vi "Get Number of Channels.vi"(8 "error in (no error)":errorcluster, 11 "Refnum in":refnum<k21>) -> (0 "error out":errorcluster, 3 "Number of Channels":i32)   [LabVIEW 2026, in "Acquisition.lvlib"]
uses:
  Acquisition.lvlib
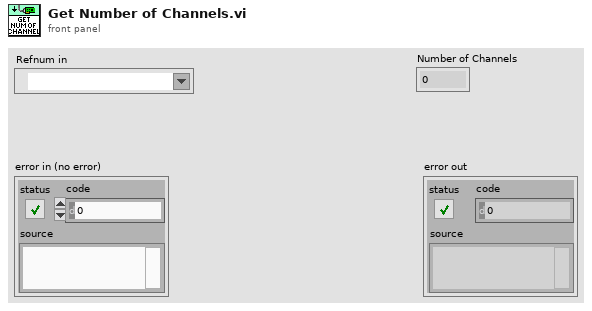
[diagram p1: front panel]
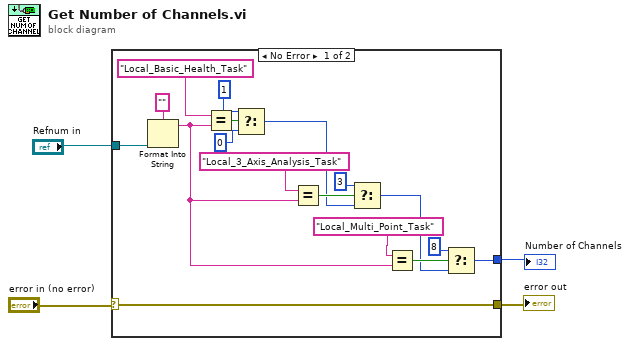
[diagram p0: block diagram]
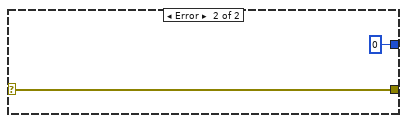
[diagram p2: hidden frame]
diagram:
  n1 = case shown="No Error" "error in (no error)" {
    selector: "error in (no error)" -> [w6 w23]
    tunnel: "Refnum in" -> [w17 _]
    tunnel: [w7 0] -> w3
    tunnel: [w6 w23] -> w1
    frame No Error {
      n2 = Format Into String(format string="", w17) -> (resulting string=w9:string)  [unwired: 2 in, 1 out]
      n3 = Equal?(x="Local_Basic_Health_Task" ("format string"), y=w9) -> (x = y?=w18:bool)
      n4 = Select(t=1, s=w18, f=0) -> (s? t:f=w13:i32)
      n5 = Equal?(x="Local_3_Axis_Analysis_Task" ("format string"), y=w9) -> (x = y?=w14:bool)
      n6 = Select(t=3, s=w14, f=w13) -> (s? t:f=w8:i32)
      n7 = Equal?(x="Local_Multi_Point_Task" ("format string"), y=w9) -> (x = y?=w11:bool)
      n8 = Select(t=8, s=w11, f=w8) -> (s? t:f=w7:i32)
    }
    frame Error {
    }
  }
  "Number of Channels" <- w3
  "error out" <- w1
